vi "Logic of Energy Detection.vi"() -> ()   [LabVIEW 2015]
uses:
  <vilib>/measure/maspectr.llb/FFT Power Spectrum and PSD for 1 Chan.vi
  <instrlib>/niUSRP/niUSRP Fetch Rx Data (CDB Cluster).vi
  <vilib>/measure/NI_MAPro.lvlib
panel:
  out "Power Spectrum / PSD":cluster{"f0":dbl, "df":dbl, "magnitude":dbl[]} {"magnitude" format="%.2p"; "f0" format="%0.2p"; "df" format="%0.2p"}
  out "SNR":dbl
  out "x/y":dbl
  in  "IQ rate":dbl=100000.0 format="%#_6p"
  in  "gain":dbl format="%#_6f"
  out "x+y":dbl
  out "CH1 is Free":bool
  out "CH2 is Free":bool
  out "CH3 is Free":bool
  out "CH4 is Free":bool
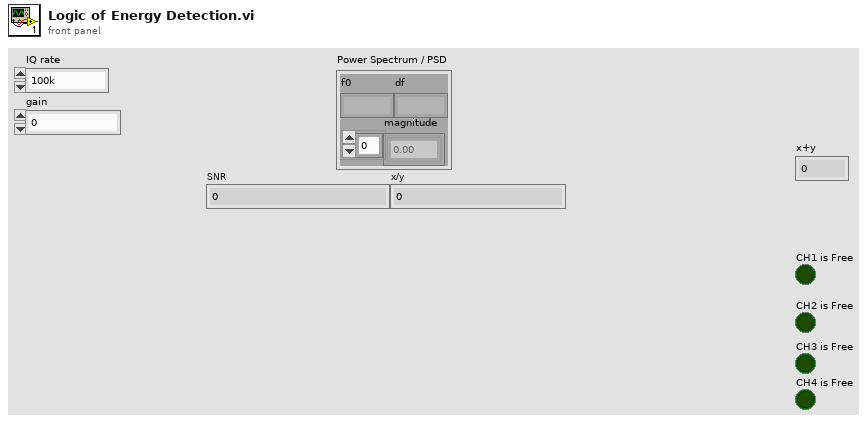
[diagram p1: front panel]
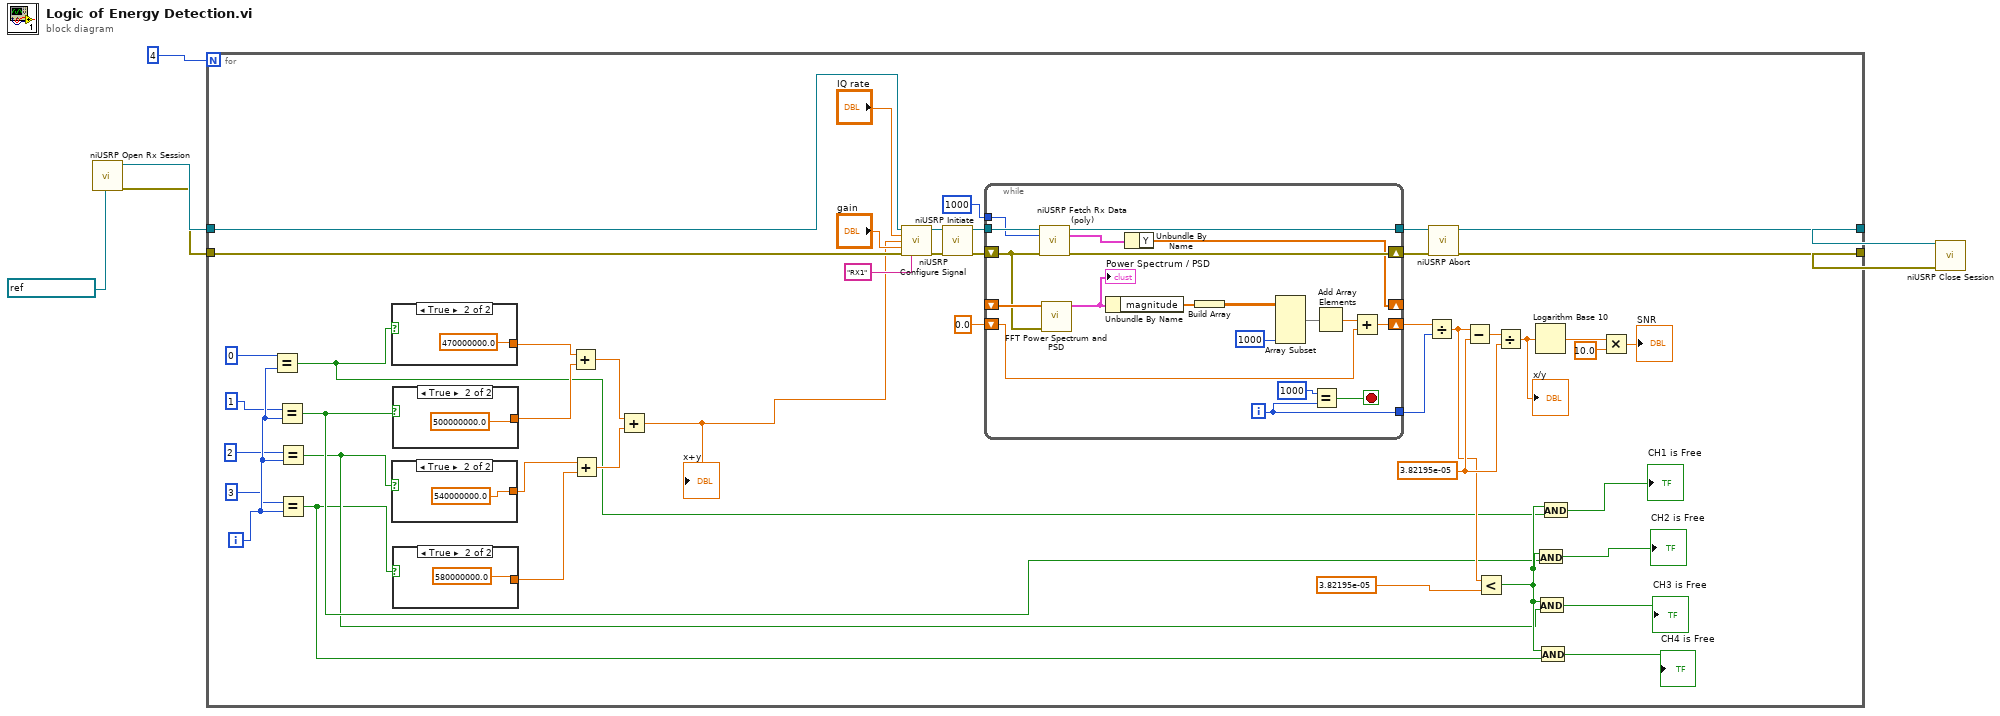
[diagram p0: block diagram]
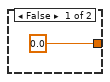
[diagram p2: hidden frame]
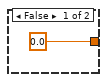
[diagram p3: hidden frame]
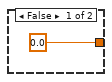
[diagram p4: hidden frame]
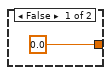
[diagram p5: hidden frame]
diagram:
  n1 = call <instrlib>:"niUSRP Open Rx Session.vi"("device names"=refnum<k15> "192.168.10.4") -> ("session handle out"=w6:refnum<k15>, "error out"=w5:errorcluster)  [unwired: 13 in]
  n2 = for {
    N: 4 -> [_]
    tunnel: w6 -> [w52]
    tunnel: w5 -> [w49]
    tunnel: [w35] -> w2
    tunnel: [w34] -> w1
    i -> [w29]
    w31 = 3.82195e-05 ("y")
    n3 = Equal?(x=0, y=w29) -> (x = y?=w14:bool)
    n4 = Equal?(x=1, y=w29) -> (x = y?=w13:bool)
    n5 = Equal?(x=2, y=w29) -> (x = y?=w12:bool)
    n6 = Equal?(x=3, y=w29) -> (x = y?=w11:bool)
    n7 = case shown="True" w14 {
      tunnel: [0.0 470000000.0] -> w24
      frame False {
      }
      frame True {
      }
    }
    n8 = case shown="True" w12 {
      tunnel: [0.0 540000000.0] -> w22
      frame False {
      }
      frame True {
      }
    }
    n9 = case shown="True" w13 {
      tunnel: [0.0 500000000.0] -> w23
      frame False {
      }
      frame True {
      }
    }
    n10 = case shown="True" w11 {
      tunnel: [0.0 580000000.0] -> w19
      frame False {
      }
      frame True {
      }
    }
    n11 = Add(x=w24, y=w23) -> (x+y=w21:dbl)
    n12 = Add(x=w22, y=w19) -> (x+y=w20:dbl)
    n13 = Add(x=w21, y=w20) -> (x+y=w16:dbl)
    "x+y" <- w16
    n14 = call <instrlib>:"niUSRP Configure Signal.vi"("session handle"=w52, "IQ rate"="IQ rate", "carrier frequency"=w16, "gain"="gain", "error in (no error)"=w49, "active antenna"="RX1") -> ("session handle out"=w51:refnum<k15>, "error out"=w50:errorcluster)  [unwired: 5 in, 3 out]
    n15 = call <instrlib>:"niUSRP Initiate.vi"("session handle"=w51, "error in (no error)"=w50) -> ("session handle out"=w48:refnum<k15>, "error out"=w47:errorcluster)  [unwired: 12 in]
    n16 = while {
      tunnel: w48 -> [w79]
      shift-right: [w63] -> w46
      shift-left: w47 -> [w76]
      tunnel: [w78] -> w45
      shift-right: [w61] -> _
      shift-left: _ -> [w77]
      shift-right: [w70] -> w43
      shift-left: 0.0 -> [w71]
      tunnel: [w65] -> w42
      tunnel: 1000 -> [w68]
      i -> [w65]
      stop <- w64 stop-if-true
      n17 = call-poly <instrlib>:"niUSRP Fetch Rx Data (poly).vi"("session handle"=w79, "number of samples"=w68, "error in (no error)"=w76) -> ("session handle out"=w78:refnum<k15>, "data"=w62:cluster{"t0":dbl, "dt":dbl, "Y":cdb[]}, "error out"=w63:errorcluster)  [unwired: 9 in, 1 out]
      n18 = call-poly <vilib>:"FFT Power Spectrum and PSD.vi"("error in (no error)"=w76, "time signal"=w77) -> ("Power Spectrum / PSD"=w75:cluster{"f0":dbl, "df":dbl, "magnitude":dbl[]})  [unwired: 6 in, 3 out]
      "Power Spectrum / PSD" <- w75
      n19 = Unbundle By Name(w75) -> ("magnitude"=w74:dbl[])
      n20 = Unbundle By Name(w62) -> ("Y"=w61:cdb[])
      n21 = Build Array(w74) -> (w73:dbl[][])
      n22 = Array Subset(array=w73, length (col)=1000 ("length")) -> (w72:dbl[][])  [unwired: 3 in]
      n23 = Equal?(x=1000, y=w65) -> (x = y?=w64:bool)
      n24 = Add Array Elements(numeric array=w72) -> (sum=w69:dbl)
      n25 = Add(x=w69, y=w71) -> (x+y=w70:dbl)
    }
    n26 = Divide(x=w43, y=w42) -> (x/y=w18:dbl)
    n27 = call <instrlib>:"niUSRP Abort.vi"("session handle"=w45, "error in (no error)"=w46) -> ("session handle out"=w35:refnum<k15>, "error out"=w34:errorcluster)  [unwired: 12 in]
    n28 = Subtract(x=w18, y=w31) -> (x-y=w30:dbl)
    n29 = Less?(x=w18, y=3.82195e-05) -> (x < y?=w15:bool)
    n30 = Divide(x=w30, y=w31) -> (x/y=w41:dbl)
    "x/y" <- w41
    n31 = Logarithm Base 10(1:w41) -> (0:w40:dbl)
    n32 = And(x=w15, y=w13) -> (x .and. y?=→"CH2 is Free":bool)
    n33 = And(x=w15, y=w12) -> (x .and. y?=→"CH3 is Free":bool)
    n34 = And(x=w15, y=w11) -> (x .and. y?=→"CH4 is Free":bool)
    n35 = And(x=w15, y=w14) -> (x .and. y?=→"CH1 is Free":bool)
    n36 = Multiply(x=w40, y=10.0) -> (x*y=→"SNR":dbl)
  }
  n37 = call <instrlib>:"niUSRP Close Session.vi"("session handle"=w2, "error in (no error)"=w1) -> ()  [unwired: 13 in, 1 out]
